vi "Launcher.vi"   [LabVIEW 2020]
uses:
  MainController/MainController.lvclass
  C:/Program Files (x86)/National Instruments/LabVIEW 2020/vi.lib/ActorFramework/Actor/Actor.lvclass
  <vilib>/ActorFramework/Actor/Actor.lvclass
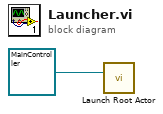
[diagram p0: block diagram]
diagram:
  n1 = call <vilib>:"Launch Root Actor.vi"("Actor"=refnum<class "MainController.lvclass"> refnum ("MainController.lvlib:MainController.lvclass")) -> ()  [unwired: 9 in, 2 out]
